vi "ReadSetting.vi"() -> ()   [LabVIEW 2013]
uses:
  <vilib>/Utility/file.llb/Read From Spreadsheet File (string).vi
  <vilib>/Utility/file.llb/Read From Spreadsheet File (DBL).vi
  Global 2.vi
panel:
  in  "Select":bool=TRUE
  in  "Filename (213)":string="TEQ3559937015.csv"
  out "Gain":dbl format="%#_13g"
  out "IFatt dB":dbl format="%#_13g"
  out "RFgen dBm":dbl format="%#_13g"
  in  "Filename (224)":string="TEQ3559748002.csv"
  out "Chan #":dbl format="%#_13g"
  out "Qamp":dbl format="%#_13g"
  out "Phase":dbl format="%#_13g"
  out "Offset":dbl format="%#_13g"
  out "Tune":dbl format="%#_13g"
  out "Nstep":dbl format="%#_13g"
  out "Fstep":dbl format="%#_13g"
  out "Array Vals":dbl[](array[numeric])
  out "Array":dbl[][](array[numeric])
  out "Text":string[][](array[string])
  out "Chars":i32
  out "Fcen":dbl format="%#_13g"
  out "File size (bytes)":i32
  out "File path":string
  # "Loader for global NMR Settings"
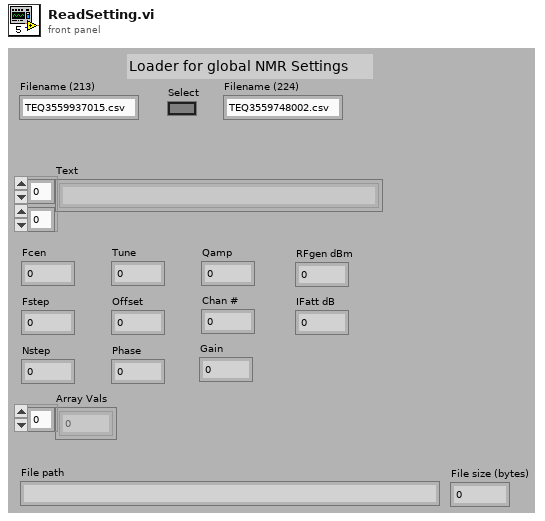
[diagram p1: front panel]
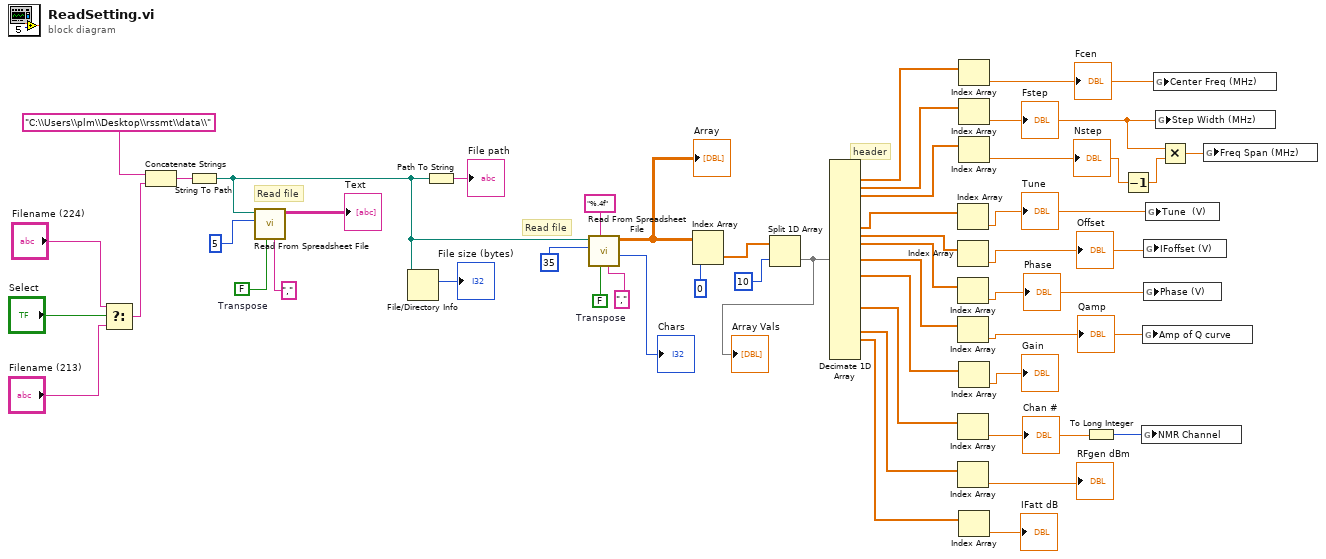
[diagram p0: block diagram]
diagram:
  w35 = FALSE  # Transpose
  w45 = FALSE  # Transpose
  # "Read file"
  # "Read file"
  # "header"
  n1 = Select(t="Filename (224)", s="Select", f="Filename (213)") -> (s? t:f=w2:string)
  n2 = Concatenate Strings "Concatenate Strings"("C:\\Users\\plm\\Desktop\\rssmt\\data\\", w2) -> (w47:string)
  n3 = String To Path(string=w47) -> (path=w37:path)
  n4 = call-poly <vilib>:"Read From Spreadsheet File.vi"("delimiter (\\t)"=",", "transpose (no:F)"=w35, "number of rows (all:-1)"=5, "file path (dialog if empty)"=w37) -> ("all rows"=→"Text":string[][])  [unwired: 3 in, 4 out]
  n5 = File/Directory Info(path=w37) -> (size=→"File size (bytes)":i64)  [unwired: 1 in, 6 out]
  n6 = Path To String(path=w37) -> (string=→"File path":string)
  n7 = call-poly <vilib>:"Read From Spreadsheet File.vi"("delimiter (\\t)"=",", "transpose (no:F)"=w45, "format (%.3f)"="%.4f", "number of rows (all:-1)"=35, "file path (dialog if empty)"=w37) -> ("mark after read (chars.)"=→"Chars":i32, "all rows"=w30:dbl[][])  [unwired: 2 in, 3 out]
  "Array" <- w30
  n8 = Index Array "Index Array"(array=w30, index (col)=0) -> (element=w29:dbl[])  [unwired: 1 in]
  n9 = Split 1D Array(array=w29, index=10) -> (second subarray=w27:dbl[])  [unwired: 1 out]
  "Array Vals" <- w27
  n10 = Decimate 1D Array(w27) -> (w41:dbl[], w40:dbl[], w39:dbl[], w26:dbl[], w25:dbl[], w24:dbl[], w23:dbl[], w17:dbl[], w22:dbl[], w19:dbl[], w18:dbl[])  [unwired: 14 out]
  n11 = Index Array(array=w26) -> (element=w15:dbl)  [unwired: 1 in]
  "Tune" <- w15
  n12 = Index Array(array=w25) -> (element=w14:dbl)  [unwired: 1 in]
  "Offset" <- w14
  n13 = Index Array(array=w24) -> (element=w13:dbl)  [unwired: 1 in]
  "Phase" <- w13
  n14 = Index Array(array=w23) -> (element=w12:dbl)  [unwired: 1 in]
  "Qamp" <- w12
  n15 = Index Array(array=w22) -> (element=w11:dbl)  [unwired: 1 in]
  "Chan #" <- w11
  n16 = Index Array(array=w19) -> (element=→"RFgen dBm":dbl)  [unwired: 1 in]
  n17 = Index Array "Index Array"(array=w41) -> (element=w9:dbl)  [unwired: 1 in]
  "Fcen" <- w9
  n18 = Index Array(array=w40) -> (element=w8:dbl)  [unwired: 1 in]
  "Fstep" <- w8
  n19 = Index Array(array=w39) -> (element=w7:dbl)  [unwired: 1 in]
  "Nstep" <- w7
  n20 = Index Array(array=w17) -> (element=→"Gain":dbl)  [unwired: 1 in]
  n21 = Index Array(array=w18) -> (element=→"IFatt dB":dbl)  [unwired: 1 in]
  n22 = To Long Integer(number=w11) -> (32bit integer=w10:i32)
  n23 = Decrement(x=w7) -> (x-1=w6:dbl)
  n24 = global write "Global 2.vi" "NMR Channel"(w10) -> ()
  n25 = global write "Global 2.vi" "Amp of Q curve"(w12) -> ()
  n26 = global write "Global 2.vi" "IFoffset (V)"(w14) -> ()
  n27 = global write "Global 2.vi" "Phase (V)"(w13) -> ()
  n28 = global write "Global 2.vi" "Tune  (V)"(w15) -> ()
  n29 = global write "Global 2.vi" "Center Freq (MHz)"(w9) -> ()
  n30 = global write "Global 2.vi" "Step Width (MHz)"(w8) -> ()
  n31 = Multiply(x=w8, y=w6) -> (x*y=w5:dbl)
  n32 = global write "Global 2.vi" "Freq Span (MHz)"(w5) -> ()
